vi "ReadVandI.vi"(8 "error in (no error)":errorcluster, 11 "axopatch-200B in":refnum<class "axopatch-200B.lvclass">) -> (0 "error out":errorcluster, 3 "axopatch-200B out":refnum<class "axopatch-200B.lvclass">)   [LabVIEW 2014, in "axopatch-200B.lvclass"]
uses:
  axopatch-200B.lvclass
  <vilib>/DAQmx/read.llb/DAQmx Read (Analog 1D DBL 1Chan NSamp).vi
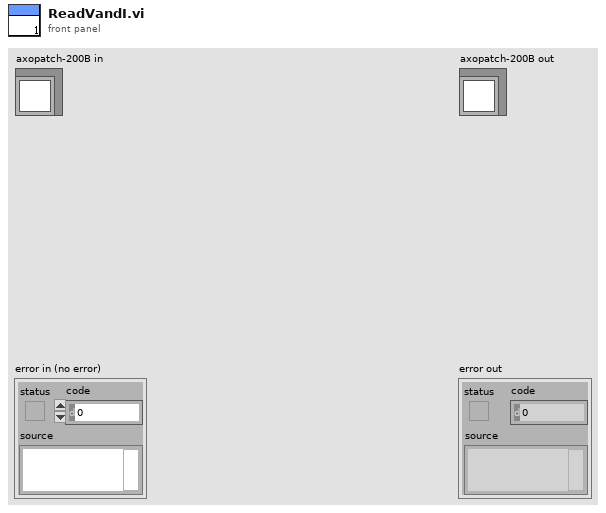
[diagram p1: front panel]
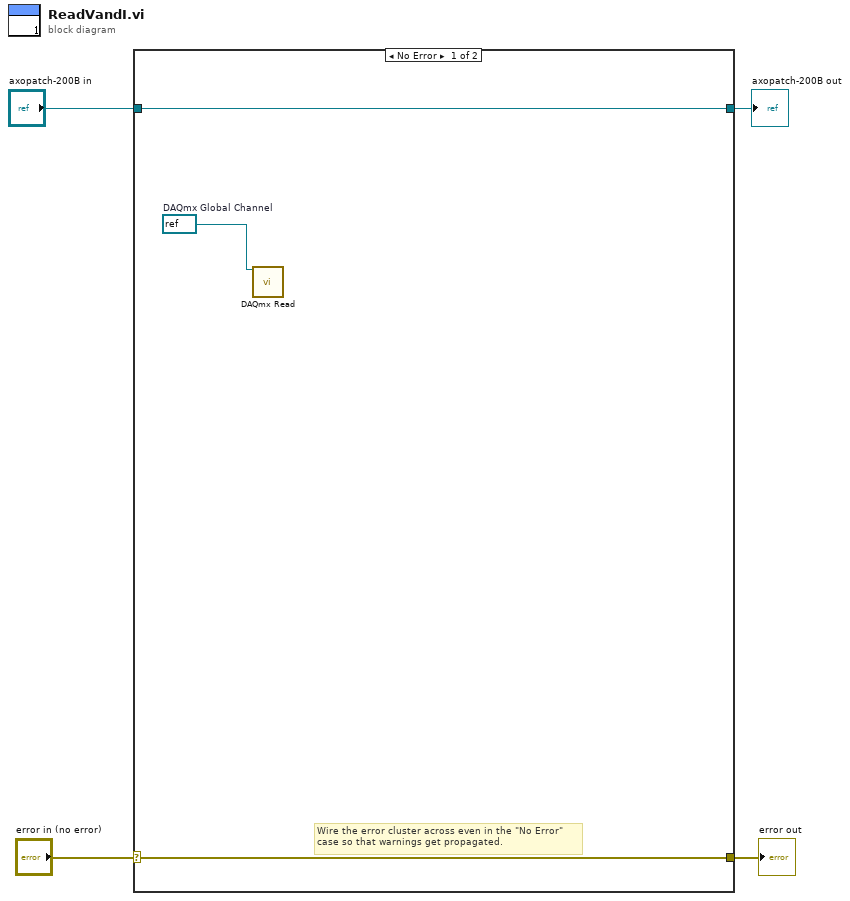
[diagram p0: block diagram]
diagram:
  n1 = case shown="No Error" "error in (no error)" {
    selector: "error in (no error)" -> [w6 w9]
    tunnel: [w6 w9] -> w3
    tunnel: [w7 w8] -> w1
    tunnel: "axopatch-200B in" -> [w7 w8]
    frame No Error {
      w5 = refnum<k21> refnum  # DAQmx Global Channel
      # "Wire the error cluster across even in the \"No Error\"\ncase so that warnings get propagated."
      n2 = call-poly <vilib>:"DAQmx Read.vi"("task/channels in"=w5) -> ()  [unwired: 12 in, 3 out]
    }
    frame Error {
    }
  }
  "error out" <- w3
  "axopatch-200B out" <- w1
